vi "Start Global Motor Values.vi"   [LabVIEW 2014]
uses:
  Global Variables.vi
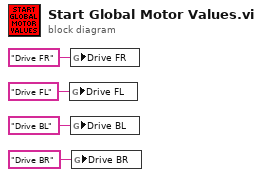
[diagram p0: block diagram]
diagram:
  n1 = global write "Global Variables.vi" "Drive FL"("Drive FL") -> ()
  n2 = global write "Global Variables.vi" "Drive FR"("Drive FR") -> ()
  n3 = global write "Global Variables.vi" "Drive BL"("Drive BL") -> ()
  n4 = global write "Global Variables.vi" "Drive BR"("Drive BR") -> ()
